vi "Suite.vi"(8 "error in (no error)":errorcluster, 11 "LUnit Test Case in":refnum<class "LUnit Test Case.lvclass">) -> (0 "error out":errorcluster, 2 "LUnit Test Suite Out":refnum<class "LUnit Test Suite.lvclass">, 3 "LUnit Test Case out":refnum<class "LUnit Test Case.lvclass">)   [LabVIEW 2020, in "LUnit Test Case.lvclass"]
uses:
  LUnit Test Case.lvclass
  C:/git/astemes-lunit/source/Core/Runnable/Runnable.lvclass
  LUnit Test Suite/LUnit Test Suite.lvclass
  LUnit Test Case.lvclass/LUnit Test Case.ctl
  <vilib>/Utility/LVClass/Get LV Class Default Value.vi
  <vilib>/Utility/LVClass/Get LV Class Name.vi
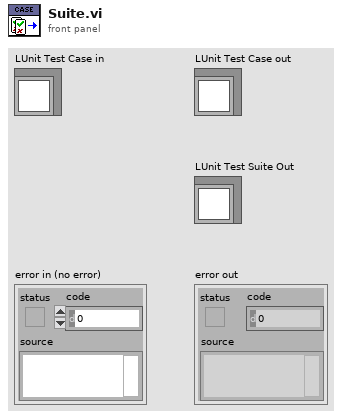
[diagram p1: front panel]
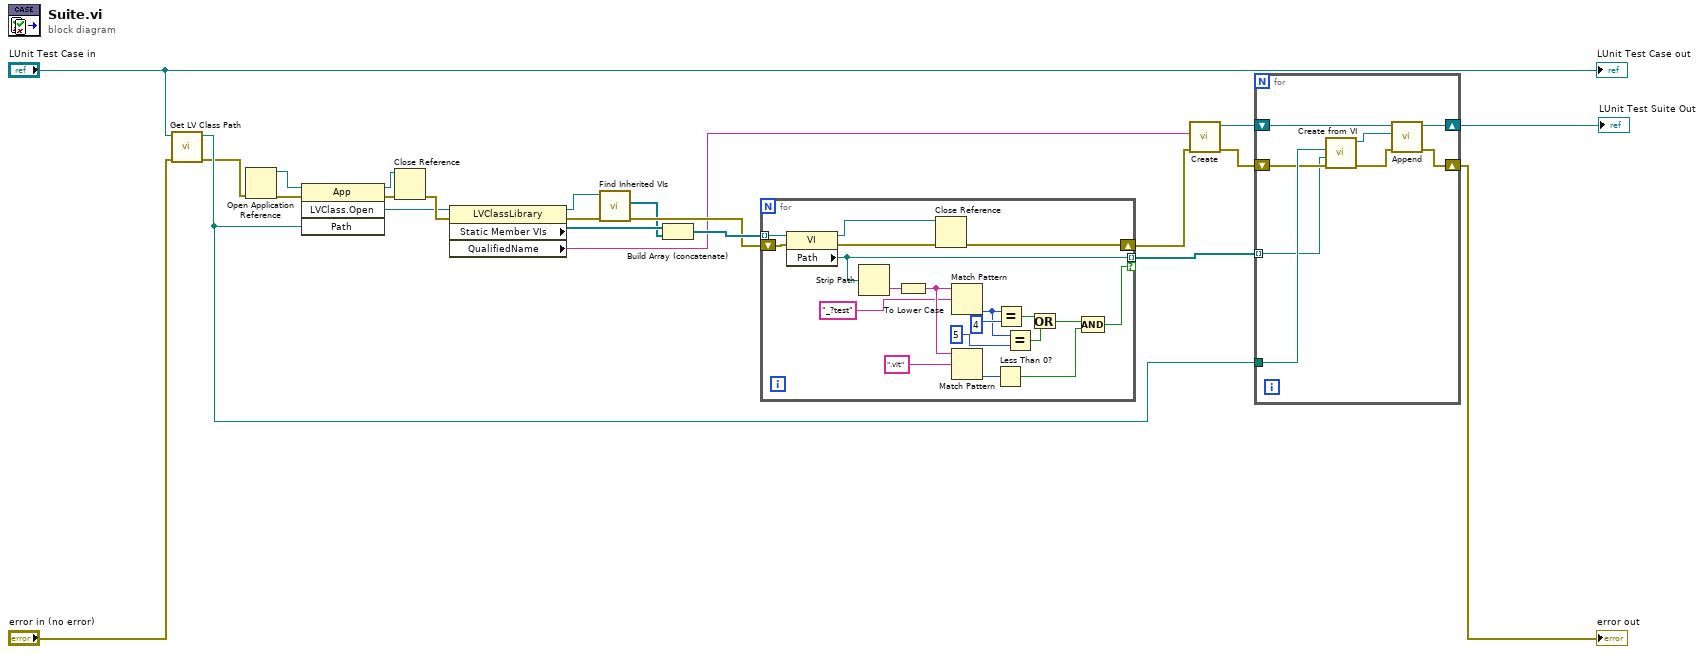
[diagram p0: block diagram]
diagram:
  n1 = call <vilib>:"Get LV Class Path.vi"("error in (no error)"="error in (no error)", "object"="LUnit Test Case in") -> ("error out"=w4:errorcluster, "class path"=w5:path)  [unwired: 8 in]
  n2 = Open Application Reference(8:w4) -> (0:w21:errorcluster, 3:w22:refnum<vi>)  [unwired: 3 in]
  n3 = invoke class="App" method="LVClass.Open"(reference=w22, error in=w21, "Path"=w5) -> (reference out=w16:refnum<vi>, error out=w20:errorcluster, "LVClass.Open"=w14:refnum<vi>)  [unwired: 1 in, 1 out]
  n4 = Close Reference(reference=w16, error in (no error)=w20) -> (error out=w17:errorcluster)
  n5 = property class="LVClassLibrary"(reference=w14, error in=w17) -> (reference out=w6:refnum<vi>, error out=w7:errorcluster, "Static Member VIs"=w19:refnum<vi>[], "QualifiedName"=w8:string)
  n6 = call "Find Inherited VIs.vi"("error in (no error)"=w7, "LVClassLibrary in"=w6) -> ("error out"=w13:errorcluster, "Inherited Dynamic Member VIs"=w12:refnum<vi>[])  [unwired: 8 in]
  n7 = Build Array (concatenate)(w19, w12) -> (w15:refnum<vi>[])
  n8 = for {
    tunnel: w15 -> [w42] mode=indexing
    tunnel: [w37] -> w18 mode=indexing if=w32
    shift-right: [w39] -> w9
    shift-left: w13 -> [w41]
    n9 = property class="VI"(reference=w42, error in=w41) -> (reference out=w38:refnum<vi>, error out=w40:errorcluster, "Path"=w37:path)
    n10 = Strip Path(path=w37) -> (name=w36:string)  [unwired: 1 out]
    n11 = To Lower Case(string=w36) -> (all lower case string=w35:string)
    n12 = Close Reference(reference=w38, error in (no error)=w40) -> (error out=w39:errorcluster)
    n13 = Match Pattern(string=w35, regular expression="_?test") -> (offset past match=w29:i32)  [unwired: 1 in, 3 out]
    n14 = Match Pattern(string=w35, regular expression=".vit") -> (offset past match=w33:i32)  [unwired: 1 in, 3 out]
    n15 = Less Than 0?(x=w33) -> (x < 0?=w31:bool)
    n16 = Equal?(x=w29, y=4) -> (x = y?=w27:bool)
    n17 = Equal?(x=w29, y=5) -> (x = y?=w24:bool)
    n18 = Or(x=w27, y=w24) -> (x .or. y?=w25:bool)
    n19 = Compound Arithmetic op=AND(w25, w31) -> (w32:bool)
  }
  n20 = call "Create.vi"("error in (no error)"=w9, "Suite Name"=w8) -> ("error out"=w10:errorcluster, "LUnit Test Suite Out"=w11:refnum<class "LUnit Test Suite.lvclass">)  [unwired: 8 in]
  n21 = for {
    tunnel: w5 -> [w50]
    tunnel: w18 -> [w44] mode=indexing
    shift-right: [w48] -> w3
    shift-left: w11 -> [w49]
    shift-right: [w46] -> w1
    shift-left: w10 -> [w45]
    n22 = call "Create from VI.vi"("error in (no error)"=w45, "Test Method VI Path"=w44, "Test Case LVCLass Path"=w50) -> ("error out"=w47:errorcluster, "LUnit Test Case Out"=w43:refnum<class "LUnit Test Case.lvclass">)  [unwired: 7 in]
    n23 = call "Append.vi"("error in (no error)"=w47, "Runnable"=w43, "LUnit Test Suite In"=w49) -> ("error out"=w46:errorcluster, "LUnit Test Suite Out"=w48:refnum<class "LUnit Test Suite.lvclass">)  [unwired: 7 in]
  }
  "error out" <- w1
  "LUnit Test Suite Out" <- w3
  "LUnit Test Case out" <- "LUnit Test Case in"
